vi "ReadSystemData.vi"(8 "error in (no error)":errorcluster, 11 "DataNotifierIn":refnum<notifier>) -> (0 "error out":errorcluster, 2 "SystemData":T1 {"SourceSelect" items=["儀器1"]}, 3 "DataNotifierIn":refnum<notifier>)   [LabVIEW 2013, in "SystemData.lvclass"]
uses:
  SystemData.lvclass
  SystemDataTypeDefine.ctl
  Generator.lvclass/Generator.lvclass
  SystemData.lvclass/SystemData.ctl
panel:
  # "以notifier包裝systemData物件的參考\n如此不論在何處只要輸入正確notifier 參考\n就可以正確提出systemData物件保存的資料"
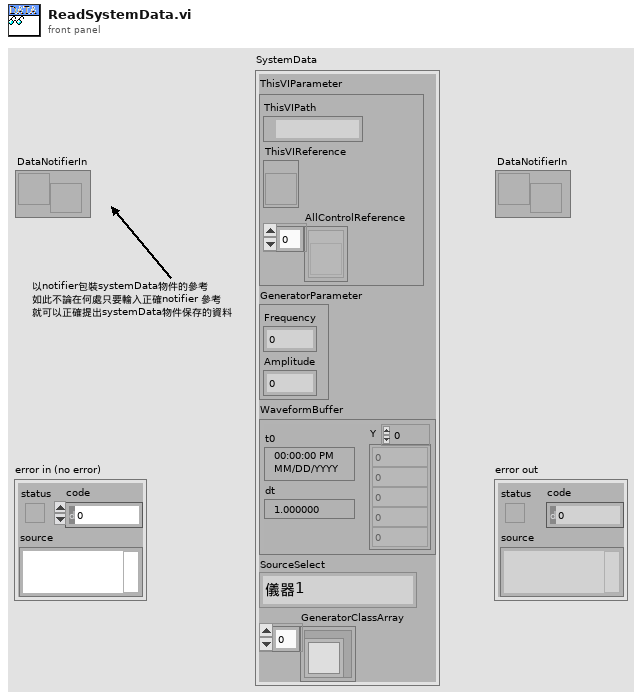
[diagram p1: front panel]
types:
  T1 = typedef "SystemData.lvclass/SystemDataTypeDefine.ctl" = cluster{"ThisVIParameter":cluster{"ThisVIPath":path, "ThisVIReference":refnum<vi>, "AllControlReference":refnum<vi>[]}, "GeneratorParameter":cluster{"Frequency":dbl, "Amplitude":dbl}, "WaveformBuffer":waveform(dbl), "SourceSelect":u16, "GeneratorClassArray":refnum<class "Generator.lvclass">[]}
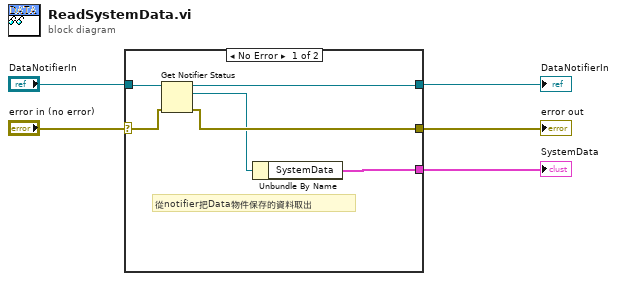
[diagram p0: block diagram]
diagram:
  n1 = case shown="No Error" "error in (no error)" {
    selector: "error in (no error)" -> [w8 w12]
    tunnel: [w7 w12] -> w4
    tunnel: [w9 w13] -> w2
    tunnel: "DataNotifierIn" -> [w10 w13]
    tunnel: [w11 _] -> w1
    frame No Error {
      # "從notifier把Data物件保存的資料取出"
      n2 = Get Notifier Status(notifier=w10, error in (no error)=w8) -> (notifier out=w9:refnum<notifier>, current notification=w6:refnum<class "SystemData.lvclass">, error out=w7:errorcluster)  [unwired: 2 out]
      n3 = Unbundle By Name(w6) -> ("SystemData"=w11:T1)
    }
    frame Error {
    }
  }
  "error out" <- w4
  "DataNotifierIn" <- w2
  "SystemData" <- w1
